vi "FTW-ActorRef-SendMessage.vi"(0 "Actor Reference":refnum<class "FTW-ActorReference.lvclass">, 5 "Message":string, 7 "Body":variant, 11 "error in":errorcluster) -> (4 "Actor Reference out":refnum<class "FTW-ActorReference.lvclass">, 15 "error out":errorcluster)   [LabVIEW 2014, in "FTW-ActorReference.lvclass"]
uses:
  FTW-ActorReference.lvclass
  Context/FTW-Actor-Context.lvclass
panel:
  # "Inputs"
  # "Outputs"
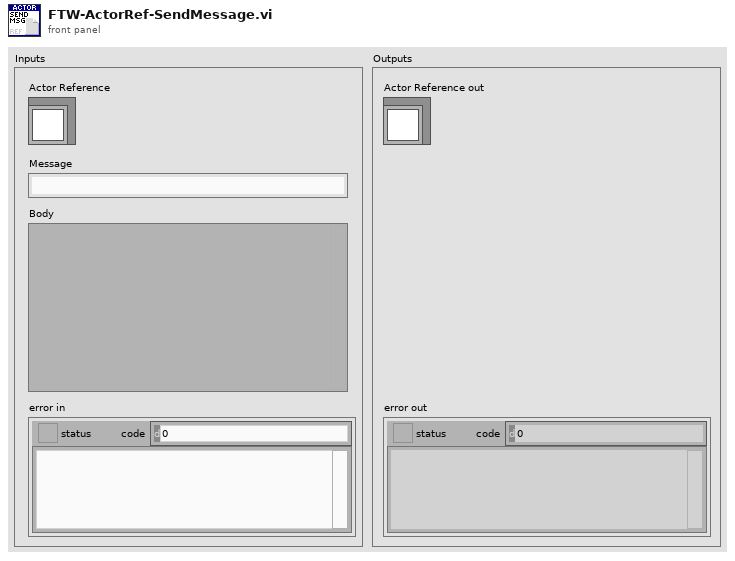
[diagram p1: front panel]
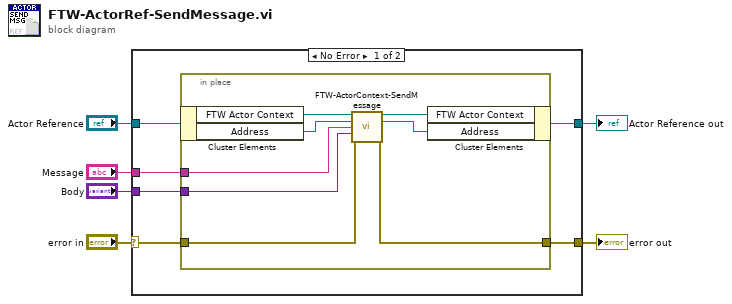
[diagram p0: block diagram]
diagram:
  n1 = case shown="No Error" "error in" {
    selector: "error in" -> [w11 w22]
    tunnel: [w9 w22] -> w5
    tunnel: "Actor Reference" -> [w12 w21]
    tunnel: [w10 w21] -> w3
    tunnel: "Message" -> [w8 _]
    tunnel: "Body" -> [w7 _]
    frame No Error {
      n2 = in-place {
        in-place-border: w11 -> [w14]
        in-place-border: [w13] -> w9
        in-place-border: w8 -> [w16]
        in-place-border: w7 -> [w15]
        n3 = in-place-cluster #1(w12) -> ("FTW Actor Context"=w20:refnum<class "FTW-Actor-Context.lvclass">, "Address"=w18:refnum<class "FTW-Actor-Address.lvclass">)
        n4 = call "FTW-ActorContext-SendMessage.vi"("Actor Reference Prototype"=w20, "FTW Actor Address"=w18, "Message"=w16, "Body"=w15, "error in"=w14) -> ("Actor Reference"=w19:refnum<class "FTW-Actor-Context.lvclass">, "FTW Actor Address out"=w17:refnum<class "FTW-Actor-Address.lvclass">, "error out"=w13:errorcluster)  [unwired: 8 in]
        n5 = in-place-cluster #1("FTW Actor Context"=w19, "Address"=w17) -> (w10:refnum<class "FTW-ActorReference.lvclass">)
      }
    }
    frame Error {
    }
  }
  "error out" <- w5
  "Actor Reference out" <- w3
